vi "G2CPU Arc Lines.vi"(6 "Auto Release (Enabled)":T1={"Auto Release Inner Radius (Enabled)"=TRUE, "Auto Release Outer Radius (Enabled)"=TRUE, "Auto Release Center X (Enabled)"=TRUE, "Auto Release Center Y (Enabled)"=TRUE, "Auto Release Stop Angle (Enabled)"=TRUE, "Auto Release Start Angle (Enabled)"=TRUE, "Auto Release Amount of Lines (Enabled)"=TRUE}, 8 "error in (no error)":errorcluster, 11 "Arc Parameters":T2) -> (0 "error out":errorcluster, 3 "Lines":T3)   [LabVIEW 2024, in "G2CPU Line Profile.lvlib"]
doc: "Create a set of points representing a set of arcs for image processing.\nThe start and stop angle is represented in radians.\n\nPoints 1 on the output define the starting point of the lines and Points 2 define the stopping point of the lines.\nThe keys put out define the grouping of the lines to each arc."
uses:
  G2CPU Line Profile.lvlib
  <vilib>/Natan Biesmans/G2CPU GPU and CPU HPC Toolkit/G2CPU Libraries/Arrays/1DArray/f32/1D Array f32.lvclass
  C:/Program Files/National Instruments/LabVIEW 2025/vi.lib/Natan Biesmans/G2CPU GPU and CPU HPC Toolkit/G2CPU Libraries/Arrays/Array/Array Prototype.lvclass
  <vilib>/Natan Biesmans/G2CPU GPU and CPU HPC Toolkit/G2CPU Libraries/Arrays/1DArray/u32/1D Array u32.lvclass
  <vilib>/Natan Biesmans/G2CPU GPU and CPU HPC Toolkit/G2CPU Libraries/Arrays/1DArray/s32/1D Array s32.lvclass
  e0e32f6f-dbee-4cf7-a23c-15f1c38ac5da.vi
  5b53b5eb-3282-4ab0-a3df-d2fdc2d889d2.vi
  6b26b44a-92c4-4941-871b-b9935c3473cd.vi
  3957dbf8-308e-4b03-8173-7c66eeded87b.vi
  caa8c30d-5c63-4e4d-bf17-3a3ad7473fd2.vi
  a4589501-e285-4deb-98d0-62cfd9af4457.vi
  d95f5dbc-a1fe-459b-be0d-cb7b5cda1adc.vi
  a5437a8b-2367-4b68-810a-8c8cff1c35d3.vi
  42a11406-5474-4d7b-b1d4-fec6161588f5.vi
  6861d397-6d08-4f02-9c31-17bd847e48c7.vi
  420c50ad-4723-4109-8ebe-d940f9fe0a85.vi
  f72864e3-a51c-4737-bd16-99c43e380a79.vi
  cfc270e5-a4f1-4f39-b466-587cd9c1b4f1.vi
  b3731f30-1c07-4127-ad91-8e9c82577051.vi
  fd436030-a523-4e7c-9b22-c56b15b39336.vi
  74647da4-d268-4f68-87d1-5e28e67c710e.vi
  e0e32f6f-dbee-4cf7-a23c-15f1c38ac5da.vi/10d88d95-1d79-457d-a71e-58ed0fd5ba1c.vi
  5b53b5eb-3282-4ab0-a3df-d2fdc2d889d2.vi/266dcd25-0bcc-42fd-b83c-a48544f38d1c.vi
  6b26b44a-92c4-4941-871b-b9935c3473cd.vi/6197f869-f6d4-49b3-9b2c-cc979b422c2e.vi
  6b26b44a-92c4-4941-871b-b9935c3473cd.vi/a7e86dbb-b4c0-485c-89c5-522e60ee265c.vi
  3957dbf8-308e-4b03-8173-7c66eeded87b.vi/6197f869-f6d4-49b3-9b2c-cc979b422c2e.vi
  3957dbf8-308e-4b03-8173-7c66eeded87b.vi/a7e86dbb-b4c0-485c-89c5-522e60ee265c.vi
  caa8c30d-5c63-4e4d-bf17-3a3ad7473fd2.vi/6197f869-f6d4-49b3-9b2c-cc979b422c2e.vi
  caa8c30d-5c63-4e4d-bf17-3a3ad7473fd2.vi/a7e86dbb-b4c0-485c-89c5-522e60ee265c.vi
  a4589501-e285-4deb-98d0-62cfd9af4457.vi/6197f869-f6d4-49b3-9b2c-cc979b422c2e.vi
  a4589501-e285-4deb-98d0-62cfd9af4457.vi/a7e86dbb-b4c0-485c-89c5-522e60ee265c.vi
  d95f5dbc-a1fe-459b-be0d-cb7b5cda1adc.vi/5793b77b-c002-4ebf-9075-685617c95341.vi
  d95f5dbc-a1fe-459b-be0d-cb7b5cda1adc.vi/2ed3ef86-c00d-4d71-b84c-20267a6dfcf9.vi
  a5437a8b-2367-4b68-810a-8c8cff1c35d3.vi/5793b77b-c002-4ebf-9075-685617c95341.vi
  a5437a8b-2367-4b68-810a-8c8cff1c35d3.vi/2ed3ef86-c00d-4d71-b84c-20267a6dfcf9.vi
  42a11406-5474-4d7b-b1d4-fec6161588f5.vi/5793b77b-c002-4ebf-9075-685617c95341.vi
  42a11406-5474-4d7b-b1d4-fec6161588f5.vi/2ed3ef86-c00d-4d71-b84c-20267a6dfcf9.vi
  6861d397-6d08-4f02-9c31-17bd847e48c7.vi/5793b77b-c002-4ebf-9075-685617c95341.vi
  6861d397-6d08-4f02-9c31-17bd847e48c7.vi/2ed3ef86-c00d-4d71-b84c-20267a6dfcf9.vi
  420c50ad-4723-4109-8ebe-d940f9fe0a85.vi/e9bebd79-1c27-4fc1-b91f-30516104c7f0.vi
  f72864e3-a51c-4737-bd16-99c43e380a79.vi/7467a0f1-0650-4e63-b635-b3d2b2ec9a4e.vi
  f72864e3-a51c-4737-bd16-99c43e380a79.vi/8ee11bc3-5ef5-497e-97f0-8db2b3aaa149.vi
  f72864e3-a51c-4737-bd16-99c43e380a79.vi/c7af9698-5e3c-4e11-95da-3024075b67d2.vi
  cfc270e5-a4f1-4f39-b466-587cd9c1b4f1.vi/a7ec311c-7cd8-4650-9526-d70ff0a769d1.vi
  b3731f30-1c07-4127-ad91-8e9c82577051.vi/e9bebd79-1c27-4fc1-b91f-30516104c7f0.vi
  fd436030-a523-4e7c-9b22-c56b15b39336.vi/7467a0f1-0650-4e63-b635-b3d2b2ec9a4e.vi
  fd436030-a523-4e7c-9b22-c56b15b39336.vi/8ee11bc3-5ef5-497e-97f0-8db2b3aaa149.vi
  fd436030-a523-4e7c-9b22-c56b15b39336.vi/c7af9698-5e3c-4e11-95da-3024075b67d2.vi
  74647da4-d268-4f68-87d1-5e28e67c710e.vi/2e03f477-51b7-4ba0-bb4f-4f838f6557e6.vi
  74647da4-d268-4f68-87d1-5e28e67c710e.vi/125d45d4-836b-469d-8a4a-6adb452f866d.vi
  74647da4-d268-4f68-87d1-5e28e67c710e.vi/8038e9ed-2e71-4568-91ba-0d873494c5ed.vi
  6b26b44a-92c4-4941-871b-b9935c3473cd.vi/6197f869-f6d4-49b3-9b2c-cc979b422c2e.vi/3e802c67-fb96-46a3-ae13-4994a8508b4f.vi
  6b26b44a-92c4-4941-871b-b9935c3473cd.vi/6197f869-f6d4-49b3-9b2c-cc979b422c2e.vi/5a50fc67-79e7-4972-80c2-92243cd53dd4.vi
  6b26b44a-92c4-4941-871b-b9935c3473cd.vi/a7e86dbb-b4c0-485c-89c5-522e60ee265c.vi/730f6c57-5c0b-4ee9-b61e-75067b25222b.vi
  6b26b44a-92c4-4941-871b-b9935c3473cd.vi/a7e86dbb-b4c0-485c-89c5-522e60ee265c.vi/096b8799-7810-404e-baca-ba9279cec4bd.vi
  6b26b44a-92c4-4941-871b-b9935c3473cd.vi/a7e86dbb-b4c0-485c-89c5-522e60ee265c.vi/0f1a5a47-bcc5-4796-ac31-8dfcfbc0d7d1.vi
  6b26b44a-92c4-4941-871b-b9935c3473cd.vi/a7e86dbb-b4c0-485c-89c5-522e60ee265c.vi/89f12e17-3330-4b72-ad8f-8dd636660732.vi
  3957dbf8-308e-4b03-8173-7c66eeded87b.vi/6197f869-f6d4-49b3-9b2c-cc979b422c2e.vi/3e802c67-fb96-46a3-ae13-4994a8508b4f.vi
  3957dbf8-308e-4b03-8173-7c66eeded87b.vi/6197f869-f6d4-49b3-9b2c-cc979b422c2e.vi/5a50fc67-79e7-4972-80c2-92243cd53dd4.vi
  3957dbf8-308e-4b03-8173-7c66eeded87b.vi/a7e86dbb-b4c0-485c-89c5-522e60ee265c.vi/730f6c57-5c0b-4ee9-b61e-75067b25222b.vi
  3957dbf8-308e-4b03-8173-7c66eeded87b.vi/a7e86dbb-b4c0-485c-89c5-522e60ee265c.vi/096b8799-7810-404e-baca-ba9279cec4bd.vi
  3957dbf8-308e-4b03-8173-7c66eeded87b.vi/a7e86dbb-b4c0-485c-89c5-522e60ee265c.vi/0f1a5a47-bcc5-4796-ac31-8dfcfbc0d7d1.vi
  3957dbf8-308e-4b03-8173-7c66eeded87b.vi/a7e86dbb-b4c0-485c-89c5-522e60ee265c.vi/89f12e17-3330-4b72-ad8f-8dd636660732.vi
  caa8c30d-5c63-4e4d-bf17-3a3ad7473fd2.vi/6197f869-f6d4-49b3-9b2c-cc979b422c2e.vi/3e802c67-fb96-46a3-ae13-4994a8508b4f.vi
  caa8c30d-5c63-4e4d-bf17-3a3ad7473fd2.vi/6197f869-f6d4-49b3-9b2c-cc979b422c2e.vi/5a50fc67-79e7-4972-80c2-92243cd53dd4.vi
  caa8c30d-5c63-4e4d-bf17-3a3ad7473fd2.vi/a7e86dbb-b4c0-485c-89c5-522e60ee265c.vi/730f6c57-5c0b-4ee9-b61e-75067b25222b.vi
  caa8c30d-5c63-4e4d-bf17-3a3ad7473fd2.vi/a7e86dbb-b4c0-485c-89c5-522e60ee265c.vi/096b8799-7810-404e-baca-ba9279cec4bd.vi
  caa8c30d-5c63-4e4d-bf17-3a3ad7473fd2.vi/a7e86dbb-b4c0-485c-89c5-522e60ee265c.vi/0f1a5a47-bcc5-4796-ac31-8dfcfbc0d7d1.vi
  caa8c30d-5c63-4e4d-bf17-3a3ad7473fd2.vi/a7e86dbb-b4c0-485c-89c5-522e60ee265c.vi/89f12e17-3330-4b72-ad8f-8dd636660732.vi
  a4589501-e285-4deb-98d0-62cfd9af4457.vi/6197f869-f6d4-49b3-9b2c-cc979b422c2e.vi/3e802c67-fb96-46a3-ae13-4994a8508b4f.vi
  a4589501-e285-4deb-98d0-62cfd9af4457.vi/6197f869-f6d4-49b3-9b2c-cc979b422c2e.vi/5a50fc67-79e7-4972-80c2-92243cd53dd4.vi
  a4589501-e285-4deb-98d0-62cfd9af4457.vi/a7e86dbb-b4c0-485c-89c5-522e60ee265c.vi/730f6c57-5c0b-4ee9-b61e-75067b25222b.vi
  a4589501-e285-4deb-98d0-62cfd9af4457.vi/a7e86dbb-b4c0-485c-89c5-522e60ee265c.vi/096b8799-7810-404e-baca-ba9279cec4bd.vi
  a4589501-e285-4deb-98d0-62cfd9af4457.vi/a7e86dbb-b4c0-485c-89c5-522e60ee265c.vi/0f1a5a47-bcc5-4796-ac31-8dfcfbc0d7d1.vi
  a4589501-e285-4deb-98d0-62cfd9af4457.vi/a7e86dbb-b4c0-485c-89c5-522e60ee265c.vi/89f12e17-3330-4b72-ad8f-8dd636660732.vi
  d95f5dbc-a1fe-459b-be0d-cb7b5cda1adc.vi/5793b77b-c002-4ebf-9075-685617c95341.vi/3e802c67-fb96-46a3-ae13-4994a8508b4f.vi
  d95f5dbc-a1fe-459b-be0d-cb7b5cda1adc.vi/5793b77b-c002-4ebf-9075-685617c95341.vi/5a50fc67-79e7-4972-80c2-92243cd53dd4.vi
  d95f5dbc-a1fe-459b-be0d-cb7b5cda1adc.vi/2ed3ef86-c00d-4d71-b84c-20267a6dfcf9.vi/730f6c57-5c0b-4ee9-b61e-75067b25222b.vi
  d95f5dbc-a1fe-459b-be0d-cb7b5cda1adc.vi/2ed3ef86-c00d-4d71-b84c-20267a6dfcf9.vi/096b8799-7810-404e-baca-ba9279cec4bd.vi
  d95f5dbc-a1fe-459b-be0d-cb7b5cda1adc.vi/2ed3ef86-c00d-4d71-b84c-20267a6dfcf9.vi/0f1a5a47-bcc5-4796-ac31-8dfcfbc0d7d1.vi
  d95f5dbc-a1fe-459b-be0d-cb7b5cda1adc.vi/2ed3ef86-c00d-4d71-b84c-20267a6dfcf9.vi/89f12e17-3330-4b72-ad8f-8dd636660732.vi
  a5437a8b-2367-4b68-810a-8c8cff1c35d3.vi/5793b77b-c002-4ebf-9075-685617c95341.vi/3e802c67-fb96-46a3-ae13-4994a8508b4f.vi
  a5437a8b-2367-4b68-810a-8c8cff1c35d3.vi/5793b77b-c002-4ebf-9075-685617c95341.vi/5a50fc67-79e7-4972-80c2-92243cd53dd4.vi
  a5437a8b-2367-4b68-810a-8c8cff1c35d3.vi/2ed3ef86-c00d-4d71-b84c-20267a6dfcf9.vi/730f6c57-5c0b-4ee9-b61e-75067b25222b.vi
  a5437a8b-2367-4b68-810a-8c8cff1c35d3.vi/2ed3ef86-c00d-4d71-b84c-20267a6dfcf9.vi/096b8799-7810-404e-baca-ba9279cec4bd.vi
  a5437a8b-2367-4b68-810a-8c8cff1c35d3.vi/2ed3ef86-c00d-4d71-b84c-20267a6dfcf9.vi/0f1a5a47-bcc5-4796-ac31-8dfcfbc0d7d1.vi
  a5437a8b-2367-4b68-810a-8c8cff1c35d3.vi/2ed3ef86-c00d-4d71-b84c-20267a6dfcf9.vi/89f12e17-3330-4b72-ad8f-8dd636660732.vi
  42a11406-5474-4d7b-b1d4-fec6161588f5.vi/5793b77b-c002-4ebf-9075-685617c95341.vi/3e802c67-fb96-46a3-ae13-4994a8508b4f.vi
  42a11406-5474-4d7b-b1d4-fec6161588f5.vi/5793b77b-c002-4ebf-9075-685617c95341.vi/5a50fc67-79e7-4972-80c2-92243cd53dd4.vi
  42a11406-5474-4d7b-b1d4-fec6161588f5.vi/2ed3ef86-c00d-4d71-b84c-20267a6dfcf9.vi/730f6c57-5c0b-4ee9-b61e-75067b25222b.vi
  42a11406-5474-4d7b-b1d4-fec6161588f5.vi/2ed3ef86-c00d-4d71-b84c-20267a6dfcf9.vi/096b8799-7810-404e-baca-ba9279cec4bd.vi
  42a11406-5474-4d7b-b1d4-fec6161588f5.vi/2ed3ef86-c00d-4d71-b84c-20267a6dfcf9.vi/0f1a5a47-bcc5-4796-ac31-8dfcfbc0d7d1.vi
  42a11406-5474-4d7b-b1d4-fec6161588f5.vi/2ed3ef86-c00d-4d71-b84c-20267a6dfcf9.vi/89f12e17-3330-4b72-ad8f-8dd636660732.vi
  6861d397-6d08-4f02-9c31-17bd847e48c7.vi/5793b77b-c002-4ebf-9075-685617c95341.vi/3e802c67-fb96-46a3-ae13-4994a8508b4f.vi
  6861d397-6d08-4f02-9c31-17bd847e48c7.vi/5793b77b-c002-4ebf-9075-685617c95341.vi/5a50fc67-79e7-4972-80c2-92243cd53dd4.vi
  6861d397-6d08-4f02-9c31-17bd847e48c7.vi/2ed3ef86-c00d-4d71-b84c-20267a6dfcf9.vi/730f6c57-5c0b-4ee9-b61e-75067b25222b.vi
  6861d397-6d08-4f02-9c31-17bd847e48c7.vi/2ed3ef86-c00d-4d71-b84c-20267a6dfcf9.vi/096b8799-7810-404e-baca-ba9279cec4bd.vi
  6861d397-6d08-4f02-9c31-17bd847e48c7.vi/2ed3ef86-c00d-4d71-b84c-20267a6dfcf9.vi/0f1a5a47-bcc5-4796-ac31-8dfcfbc0d7d1.vi
  6861d397-6d08-4f02-9c31-17bd847e48c7.vi/2ed3ef86-c00d-4d71-b84c-20267a6dfcf9.vi/89f12e17-3330-4b72-ad8f-8dd636660732.vi
  74647da4-d268-4f68-87d1-5e28e67c710e.vi/2e03f477-51b7-4ba0-bb4f-4f838f6557e6.vi/d8e2d9cc-c923-495e-b121-b6b84788c73f.vi
  74647da4-d268-4f68-87d1-5e28e67c710e.vi/2e03f477-51b7-4ba0-bb4f-4f838f6557e6.vi/345e91f0-9a5e-4de4-af9c-133346717e4a.vi
  <vilib>/Natan Biesmans/G2CPU GPU and CPU HPC Toolkit/G2CPU Libraries/Arrays/2DArray/f32/2D Array f32.lvclass
  <vilib>/Natan Biesmans/G2CPU GPU and CPU HPC Toolkit/G2CPU Libraries/Arrays/2DArray/binary/2D Array binary.lvclass
  <vilib>/Natan Biesmans/G2CPU GPU and CPU HPC Toolkit/G2CPU Libraries/Arrays/1DArray/binary/1D Array binary.lvclass
  <vilib>/Natan Biesmans/G2CPU GPU and CPU HPC Toolkit/G2CPU Libraries/Arrays/2DArray/u32/2D Array u32.lvclass
  <vilib>/Natan Biesmans/G2CPU GPU and CPU HPC Toolkit/G2CPU Libraries/Arrays/Array/G2CPU Lock Array.vi
  <vilib>/Natan Biesmans/G2CPU GPU and CPU HPC Toolkit/G2CPU Libraries/Arrays/Array/G2CPU Get Array Pointer.vi
  <vilib>/Natan Biesmans/G2CPU GPU and CPU HPC Toolkit/ArrayFire Driver/VIs/cos.vi
  <vilib>/Natan Biesmans/G2CPU GPU and CPU HPC Toolkit/G2CPU Libraries/Arrays/Array/G2CPU Set Array Pointer.vi
  <vilib>/Natan Biesmans/G2CPU GPU and CPU HPC Toolkit/G2CPU Libraries/Arrays/Array/G2CPU Unlock Array.vi
  <vilib>/Natan Biesmans/G2CPU GPU and CPU HPC Toolkit/ArrayFire Driver/VIs/sin.vi
  <vilib>/Natan Biesmans/G2CPU GPU and CPU HPC Toolkit/G2CPU Libraries/Arrays/SubVI/Lock Arrays.vi
  <vilib>/Natan Biesmans/G2CPU GPU and CPU HPC Toolkit/G2CPU Libraries/Arrays/SubVI/is 2D.vi
  <vilib>/Natan Biesmans/G2CPU GPU and CPU HPC Toolkit/ArrayFire Driver/VIs/mul.vi
  <vilib>/Natan Biesmans/G2CPU GPU and CPU HPC Toolkit/ArrayFire Driver/VIs/add.vi
  <vilib>/Natan Biesmans/G2CPU GPU and CPU HPC Toolkit/ArrayFire Driver/VIs/transpose.vi
  <vilib>/Natan Biesmans/G2CPU GPU and CPU HPC Toolkit/ArrayFire Driver/VIs/flat.vi
  <vilib>/Natan Biesmans/G2CPU GPU and CPU HPC Toolkit/ArrayFire Driver/VIs/where.vi
  <vilib>/Natan Biesmans/G2CPU GPU and CPU HPC Toolkit/ArrayFire Driver/VIs/cast.vi
  <vilib>/Natan Biesmans/G2CPU GPU and CPU HPC Toolkit/ArrayFire Driver/VIs/lookup.vi
  <vilib>/Natan Biesmans/G2CPU GPU and CPU HPC Toolkit/G2CPU Libraries/Arrays/Array/Array Prototype.lvclass
  <vilib>/Natan Biesmans/G2CPU GPU and CPU HPC Toolkit/G2CPU Libraries/Arrays/DataTypes/f32/f32.lvclass
  <vilib>/Natan Biesmans/G2CPU GPU and CPU HPC Toolkit/G2CPU Libraries/Arrays/2DArray/2D Array Prototype.lvclass
  <vilib>/Natan Biesmans/G2CPU GPU and CPU HPC Toolkit/G2CPU Libraries/Arrays/1DArray/1D Array Prototype.lvclass
  <vilib>/Natan Biesmans/G2CPU GPU and CPU HPC Toolkit/G2CPU Libraries/Arrays/DataTypes/Boolean/Boolean.lvclass
  <vilib>/Natan Biesmans/G2CPU GPU and CPU HPC Toolkit/G2CPU Libraries/Arrays/DataTypes/U32/U32.lvclass
  <vilib>/Natan Biesmans/G2CPU GPU and CPU HPC Toolkit/G2CPU Libraries/Arrays/DataTypes/I32/s32.lvclass
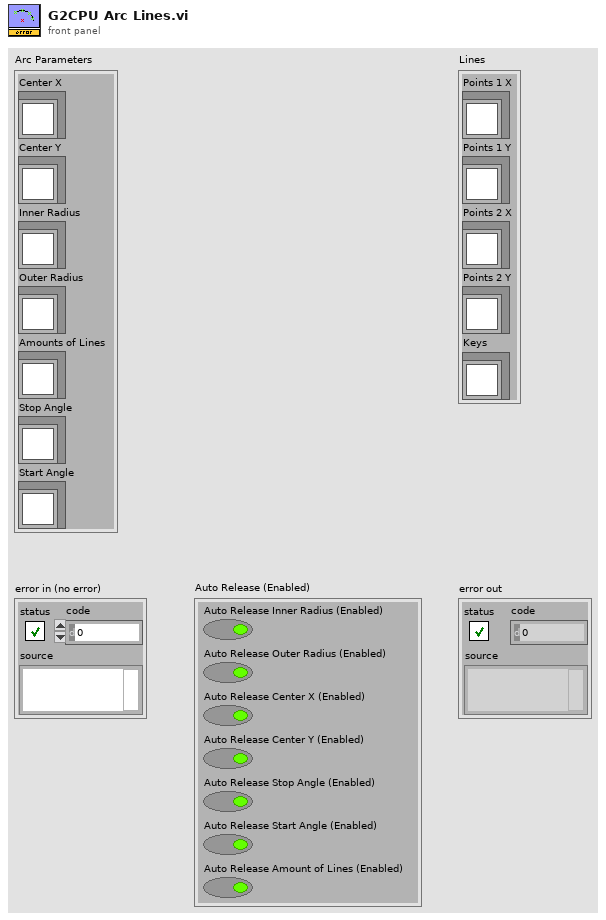
[diagram p1: front panel]
types:
  T1 = cluster{"Auto Release Inner Radius (Enabled)":bool, "Auto Release Outer Radius (Enabled)":bool, "Auto Release Center X (Enabled)":bool, "Auto Release Center Y (Enabled)":bool, "Auto Release Stop Angle (Enabled)":bool, "Auto Release Start Angle (Enabled)":bool, "Auto Release Amount of Lines (Enabled)":bool}
  T2 = cluster{"Center X":refnum<class "1D Array f32.lvclass">, "Center Y":refnum<class "1D Array f32.lvclass">, "Inner Radius":refnum<class "1D Array f32.lvclass">, "Outer Radius":refnum<class "1D Array f32.lvclass">, "Amounts of Lines":refnum<class "1D Array s32.lvclass">, "Stop Angle":refnum<class "1D Array f32.lvclass">, "Start Angle":refnum<class "1D Array f32.lvclass">}
  T3 = cluster{"Points 1 X":refnum<class "1D Array f32.lvclass">, "Points 1 Y":refnum<class "1D Array f32.lvclass">, "Points 2 X":refnum<class "1D Array f32.lvclass">, "Points 2 Y":refnum<class "1D Array f32.lvclass">, "Keys":refnum<class "1D Array u32.lvclass">}
  T4 = cluster{"Px 1":refnum<class "1D Array f32.lvclass">, "Py 1":refnum<class "1D Array f32.lvclass">, "Px 2":refnum<class "1D Array f32.lvclass">, "Py 2":refnum<class "1D Array f32.lvclass">, "Keys":refnum<class "1D Array u32.lvclass">}
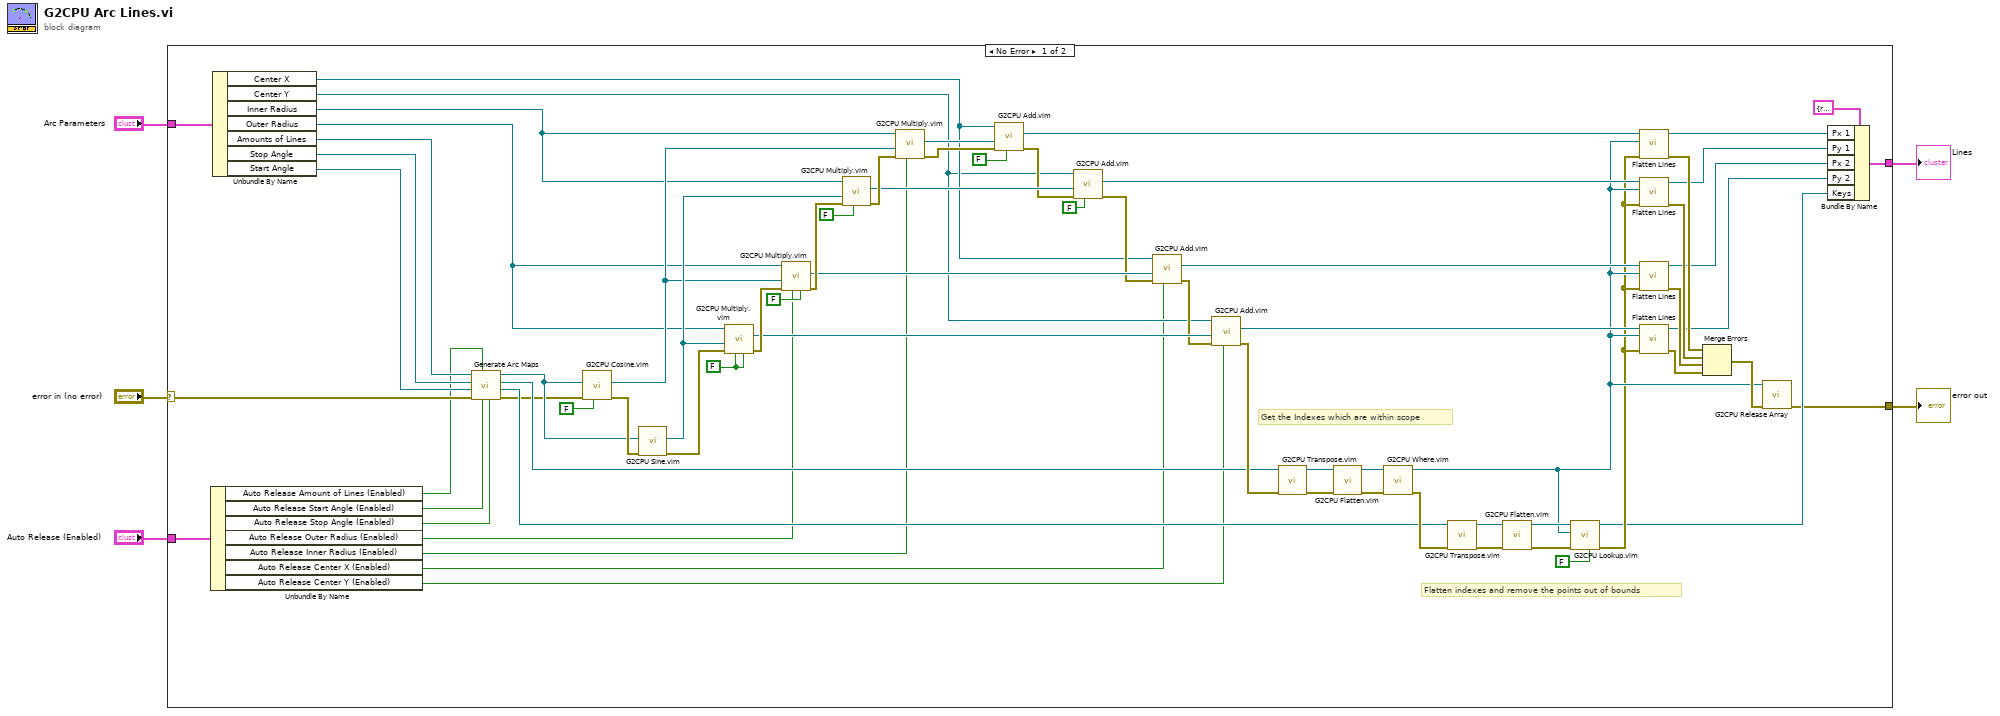
[diagram p0: block diagram]
diagram:
  n1 = case shown="No Error" "error in (no error)" {
    selector: "error in (no error)" -> [w22 w78]
    tunnel: [w33 _] -> w4
    tunnel: [w27 w78] -> w3
    tunnel: "Arc Parameters" -> [w21 _]
    tunnel: "Auto Release (Enabled)" -> [w13 _]
    frame No Error {
      w70 = FALSE ("Auto Release lhs")
      # "Flatten indexes and remove the points out of bounds"
      # "Get the Indexes which are within scope"
      n2 = Unbundle By Name(w13) -> ("Auto Release Amount of Lines (Enabled)"=w12:bool, "Auto Release Start Angle (Enabled)"=w11:bool, "Auto Release Stop Angle (Enabled)"=w10:bool, "Auto Release Outer Radius (Enabled)"=w6:bool, "Auto Release Inner Radius (Enabled)"=w7:bool, "Auto Release Center X (Enabled)"=w8:bool, "Auto Release Center Y (Enabled)"=w9:bool)
      n3 = Unbundle By Name(w21) -> ("Center X"=w20:refnum<class "1D Array f32.lvclass">, "Center Y"=w19:refnum<class "1D Array f32.lvclass">, "Inner Radius"=w18:refnum<class "1D Array f32.lvclass">, "Outer Radius"=w17:refnum<class "1D Array f32.lvclass">, "Amounts of Lines"=w16:refnum<class "1D Array s32.lvclass">, "Stop Angle"=w15:refnum<class "1D Array f32.lvclass">, "Start Angle"=w14:refnum<class "1D Array f32.lvclass">)
      n4 = call "Generate Arc Maps.vi"("Auto Release Stop Angle (Enabled)"=w10, "Auto Release Start Angle (Enabled)"=w11, "Auto Release Amount of Lines (Enabled)"=w12, "error in (no error)"=w22, "Stop Angle"=w14, "Start Angle"=w15, "Amount of Lines"=w16) -> ("error out"=w23:errorcluster, "Keys"=w24:refnum<class "2D Array u32.lvclass">, "Point mask within bounds"=w25:refnum<class "2D Array binary.lvclass">, "Arc Scales"=w26:refnum<class "2D Array f32.lvclass">)  [unwired: 1 in]
      n5 = call "G2CPU Cosine.vim"("Auto Release (Enabled)"=FALSE, "error in (no error)"=w23, "Array in"=w26) -> ("error out"=w77:errorcluster, "Array Result"=w74:refnum<class "2D Array f32.lvclass">)  [unwired: 7 in]
      n6 = call "G2CPU Sine.vim"("error in (no error)"=w77, "Array in"=w26) -> ("error out"=w73:errorcluster, "Array Result"=w75:refnum<class "2D Array f32.lvclass">)  [unwired: 8 in]
      n7 = call "G2CPU Multiply.vim"("Auto Release rhs"=w70, "Auto Release lhs"=w70, "error in (no error)"=w73, "Array rhs"=w75, "Array lhs"=w17) -> ("error out"=w72:errorcluster, "Array Result"=w63:refnum<class "2D Array f32.lvclass">)  [unwired: 5 in]
      n8 = call "G2CPU Multiply.vim"("Auto Release rhs"=FALSE, "Auto Release lhs"=w6, "error in (no error)"=w72, "Array rhs"=w74, "Array lhs"=w17) -> ("error out"=w71:errorcluster, "Array Result"=w64:refnum<class "2D Array f32.lvclass">)  [unwired: 5 in]
      n9 = call "G2CPU Multiply.vim"("Auto Release lhs"=FALSE, "error in (no error)"=w71, "Array rhs"=w75, "Array lhs"=w18) -> ("error out"=w67:errorcluster, "Array Result"=w65:refnum<class "2D Array f32.lvclass">)  [unwired: 6 in]
      n10 = call "G2CPU Multiply.vim"("Auto Release lhs"=w7, "error in (no error)"=w67, "Array rhs"=w74, "Array lhs"=w18) -> ("error out"=w62:errorcluster, "Array Result"=w66:refnum<class "2D Array f32.lvclass">)  [unwired: 6 in]
      n11 = call "G2CPU Add.vim"("Auto Release lhs (Enabled)"=FALSE, "error in (no error)"=w62, "Array rhs"=w66, "Array lhs"=w20) -> ("error out"=w61:errorcluster, "Array Result"=w53:refnum<class "2D Array f32.lvclass">)  [unwired: 6 in]
      n12 = call "G2CPU Add.vim"("Auto Release lhs (Enabled)"=FALSE, "error in (no error)"=w61, "Array rhs"=w65, "Array lhs"=w19) -> ("error out"=w60:errorcluster, "Array Result"=w54:refnum<class "2D Array f32.lvclass">)  [unwired: 6 in]
      n13 = call "G2CPU Add.vim"("Auto Release lhs (Enabled)"=w8, "error in (no error)"=w60, "Array rhs"=w64, "Array lhs"=w20) -> ("error out"=w59:errorcluster, "Array Result"=w55:refnum<class "2D Array f32.lvclass">)  [unwired: 6 in]
      n14 = call "G2CPU Add.vim"("Auto Release lhs (Enabled)"=w9, "error in (no error)"=w59, "Array rhs"=w63, "Array lhs"=w19) -> ("error out"=w35:errorcluster, "Array Result"=w56:refnum<class "2D Array f32.lvclass">)  [unwired: 6 in]
      n15 = call "G2CPU Transpose.vim"("error in (no error)"=w35, "Array In"=w25) -> ("error out"=w41:errorcluster, "Array out"=w51:refnum<class "2D Array binary.lvclass">)  [unwired: 8 in]
      n16 = call "G2CPU Flatten.vim"("error in (no error)"=w41, "Array In"=w51) -> ("error out"=w40:errorcluster, "Array out"=w50:refnum<class "1D Array binary.lvclass">)  [unwired: 8 in]
      n17 = call "G2CPU Where.vim"("error in (no error)"=w40, "Array in"=w50) -> ("error out"=w37:errorcluster, "Non Zero Indices"=w42:refnum<class "1D Array u32.lvclass">)  [unwired: 8 in]
      n18 = call "G2CPU Transpose.vim"("error in (no error)"=w37, "Array In"=w24) -> ("error out"=w39:errorcluster, "Array out"=w52:refnum<class "2D Array u32.lvclass">)  [unwired: 8 in]
      n19 = call "G2CPU Flatten.vim"("error in (no error)"=w39, "Array In"=w52) -> ("error out"=w38:errorcluster, "Array out"=w48:refnum<class "1D Array u32.lvclass">)  [unwired: 8 in]
      n20 = call "G2CPU Lookup.vim"("Auto Release Indices (Enabled)"=FALSE, "error in (no error)"=w38, "Indices (1D)"=w42, "Array In"=w48) -> ("error out"=w36:errorcluster, "Indexed Array"=w28:refnum<class "1D Array u32.lvclass">)  [unwired: 6 in]
      n21 = call "Flatten Lines.vi"("error in (no error)"=w36, "Valid Point Indexes (flattened)"=w42, "Lines In"=w53) -> ("error out"=w47:errorcluster, "Flattened Lines Out"=w32:refnum<class "1D Array f32.lvclass">)  [unwired: 7 in]
      n22 = call "Flatten Lines.vi"("error in (no error)"=w36, "Valid Point Indexes (flattened)"=w42, "Lines In"=w54) -> ("error out"=w46:errorcluster, "Flattened Lines Out"=w31:refnum<class "1D Array f32.lvclass">)  [unwired: 7 in]
      n23 = call "Flatten Lines.vi"("error in (no error)"=w36, "Valid Point Indexes (flattened)"=w42, "Lines In"=w55) -> ("error out"=w45:errorcluster, "Flattened Lines Out"=w30:refnum<class "1D Array f32.lvclass">)  [unwired: 7 in]
      n24 = call "Flatten Lines.vi"("error in (no error)"=w36, "Valid Point Indexes (flattened)"=w42, "Lines In"=w56) -> ("error out"=w44:errorcluster, "Flattened Lines Out"=w29:refnum<class "1D Array f32.lvclass">)  [unwired: 7 in]
      n25 = Merge Errors(w47, w46, w45, w44) -> (w43:errorcluster)
      n26 = call <vilib>:"G2CPU Release Array.vi"("error in (no error)"=w43, "Array in"=w42) -> ("error out"=w27:errorcluster)  [unwired: 9 in]
      n27 = Bundle By Name(cluster=T4 {"Px 1"=refnum, "Py 1"=refnum, "Px 2"=refnum, "Py 2"=refnum, "Keys"=refnum} ("Cluster"), "Px 1"=w32, "Py 1"=w31, "Px 2"=w30, "Py 2"=w29, "Keys"=w28) -> (w33:T4)
    }
    frame Error {
    }
  }
  "Lines" <- w4
  "error out" <- w3
